vi "Slack User Demo.vi"() -> ()   [LabVIEW 2015]
panel:
  out "name":string
  in  "Add Button 2":bool
  out "Workspace":string
  in  "Add Button":bool
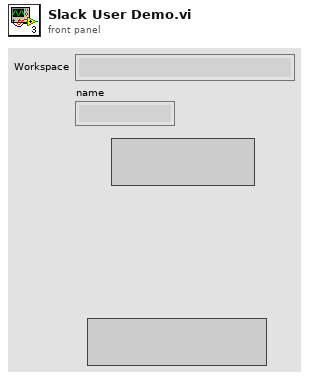
[diagram p1: front panel]
types:
  T1 = typedef "Slack-Configuration.ctl" = cluster{"app_id":string, "authed_user":cluster{"id":string}, "access_token":string, "bot_user_id":string, "team":cluster{"id":string, "name":string}, "bot channel":cluster{"id":string, "name":string}, "bot_user_name":string}
  T2 = typedef "Slack-User.ctl" = cluster{"id":string, "name":string}
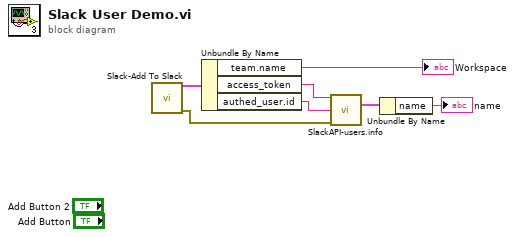
[diagram p0: block diagram]
diagram:
  n1 = call "Slack-Add To Slack.vi"() -> ("config"=w6:T1, "error out"=w4:errorcluster)  [unwired: 14 in]
  n2 = Unbundle By Name(w6) -> ("team.name"=→"Workspace":string, "access_token"=w5:string, "authed_user.id"=w3:string)
  n3 = call "SlackAPI-users.info.vi"("token"=w5, "user"=w3, "error in (no error)"=w4) -> ("user"=w2:T2)  [unwired: 10 in, 2 out]
  n4 = Unbundle By Name(w2) -> ("name"=→"name":string)
